vi "mao03.vi"() -> ()   [LabVIEW 2014]
panel:
  out "Waveform Graph 2":dynamicdata(graph)
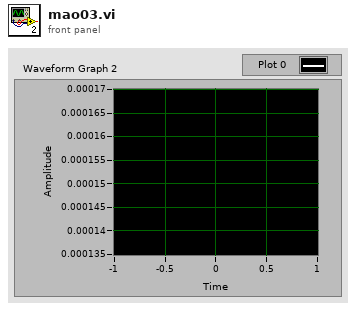
[diagram p1: front panel]
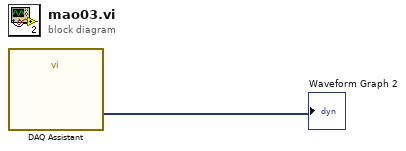
[diagram p0: block diagram]
diagram:
  n1 = call "DAQ Assistant"() -> ("data"=→"Waveform Graph 2":dynamicdata)  [unwired: 17 in, 2 out]
